vi "Reactor Write Client.vi"() -> ()   [LabVIEW 2017]
uses:
  <vilib>/OPCUA/controls/Write Status.ctl
  <vilib>/OPCUA/controls/NodeId.ctl
  <vilib>/OPCUA/client/Multiple Write Double Array.vi
  <vilib>/OPCUA/client/Multiple Write Bool Array.vi
  <vilib>/OPCUA/NI OPC UA Client.lvlib
panel:
  in  "error in (no error)":errorcluster
  in  "Stop Reactor Digital Control":bool
  in  "Node Status":T1 items=["Good"=0, "Uncertain_InitialValue"=1083310080, "Uncertain_LastUsableValue"=1083179008, "Uncertain_SensorNotAccurate"=1083375616, "Uncertain_EngineeringUnitsExceeded"=1083441152, "Bad_NoCommunication"=2150694912, "Bad_NotReadable"=2151284736, "Bad_NotWritable"=2151350272, "Bad_OutOfRange"=2151415808, "Bad_WaitingForInitialData"=2150760448]
  in  "Time Stamp":timestamp
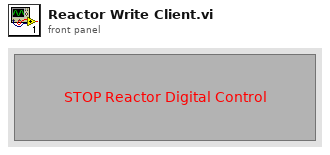
[diagram p1: front panel]
types:
  T1 = typedef "Write Status.ctl" = u32
  T2 = cluster{"message mode":enum16{"None", "Sign", "Sign and Encrypt"}, "security":enum16{"Basic256", "Basic128Rsa15"}}
  T3 = typedef "OPC UA Client Refnum.ctl" = refnum<k21>
  T4 = typedef "NodeId.ctl" = string
  T5 = cluster{"node ID":T4, "value":bool[], "timestamp (current time)":timestamp, "node status":T1}
  T6 = cluster{"node ID":T4, "value":dbl[], "timestamp (current time)":timestamp, "node status":T1}
  T7 = cluster{"node ID":T4, "value":dbl[], "timestamp (current time)":timestamp, "node status":T1}[]
  T8 = cluster{"node ID":T4, "value":bool[], "timestamp (current time)":timestamp, "node status":T1}[]
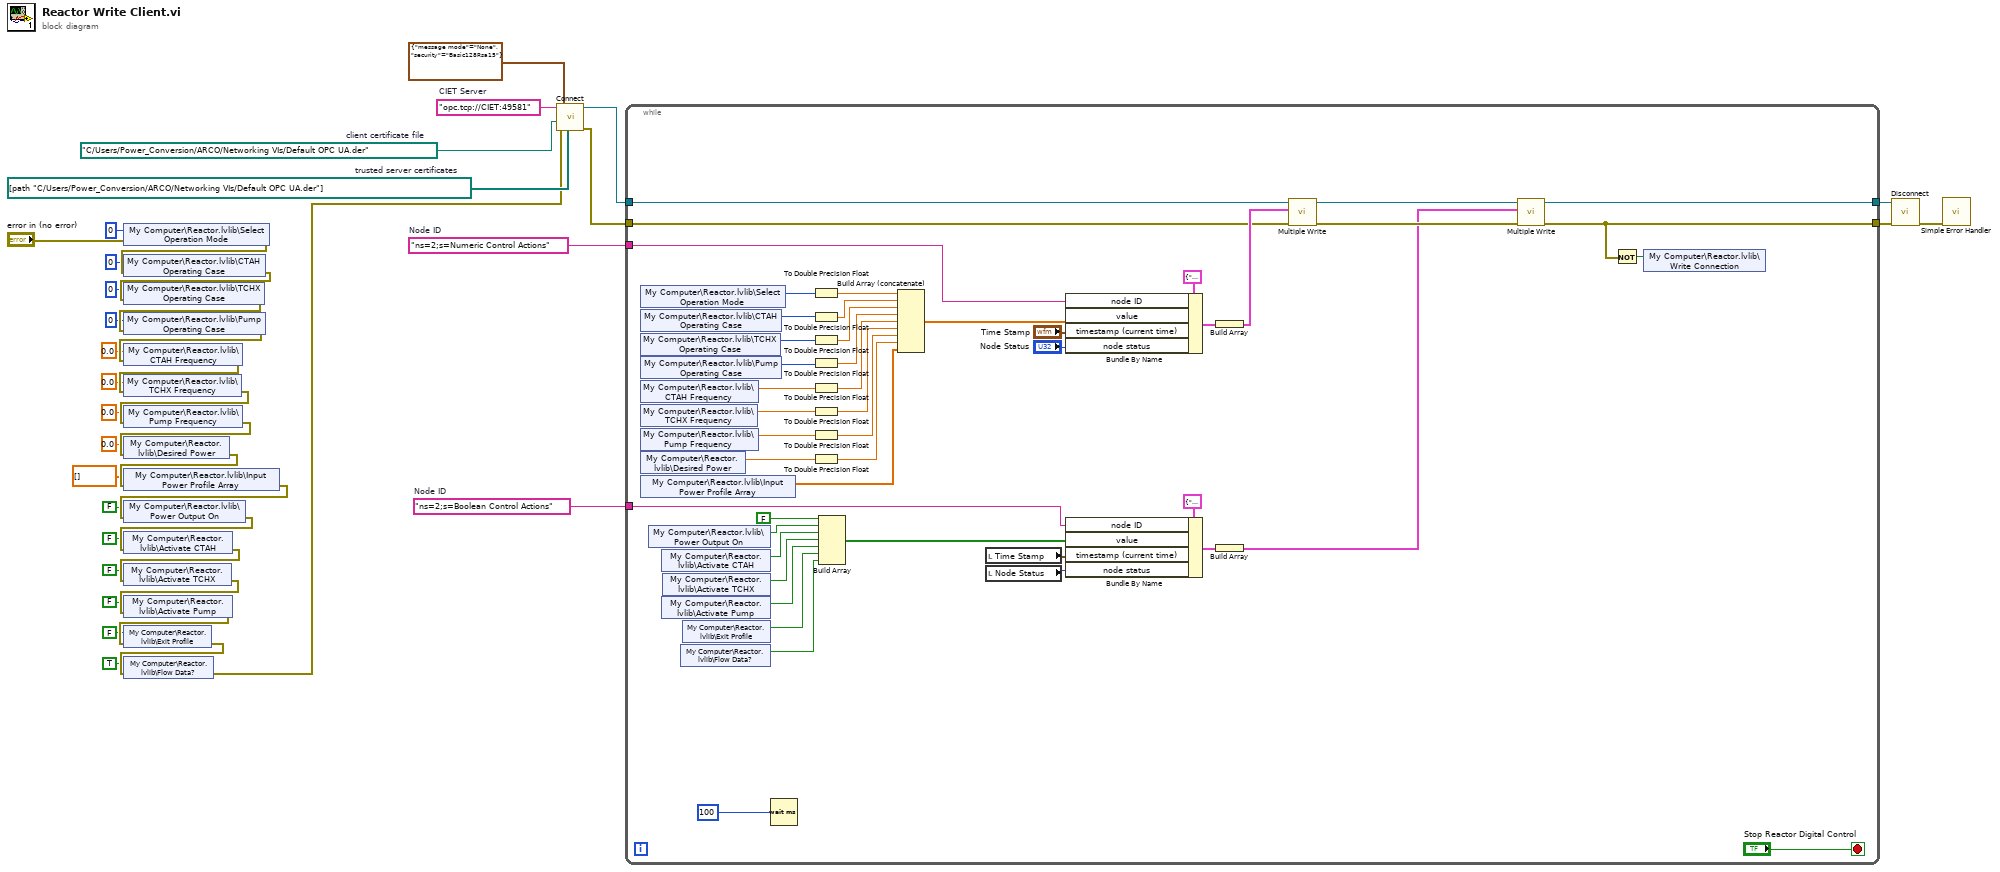
[diagram p0: block diagram]
diagram:
  w35 = "ns=2;s=Boolean Control Actions"  # Node ID
  w36 = "ns=2;s=Numeric Control Actions"  # Node ID
  w39 = path[] [path "C:/Users/Power_Conversion/ARCO/Networking VIs/Default OPC UA.der"]  # trusted server certificates
  w40 = path "C:/Users/Power_Conversion/ARCO/Networking VIs/Default OPC UA.der"  # client certificate file
  w42 = "opc.tcp://CIET:49581"  # CIET Server
  n1 = shared-variable "My Computer\\Reactor.lvlib\\Select Operation Mode"(u16 0 ("Select Operation Mode"), error in="error in (no error)") -> (error out=w30:errorcluster)
  n2 = shared-variable "My Computer\\Reactor.lvlib\\CTAH Operating Case"(0 ("CTAH Operating Case"), error in=w30) -> (error out=w29:errorcluster)
  n3 = shared-variable "My Computer\\Reactor.lvlib\\TCHX Operating Case"(0 ("TCHX Operating Case"), error in=w29) -> (error out=w28:errorcluster)
  n4 = shared-variable "My Computer\\Reactor.lvlib\\Pump Operating Case"(0 ("Pump Operating Case"), error in=w28) -> (error out=w27:errorcluster)
  n5 = shared-variable "My Computer\\Reactor.lvlib\\CTAH Frequency"(sgl 0.0 ("CTAH Frequency"), error in=w27) -> (error out=w26:errorcluster)
  n6 = shared-variable "My Computer\\Reactor.lvlib\\TCHX Frequency"(sgl 0.0 ("TCHX Frequency"), error in=w26) -> (error out=w25:errorcluster)
  n7 = shared-variable "My Computer\\Reactor.lvlib\\Pump Frequency"(sgl 0.0 ("Pump Frequency"), error in=w25) -> (error out=w24:errorcluster)
  n8 = shared-variable "My Computer\\Reactor.lvlib\\Desired Power"(sgl 0.0 ("Desired Power"), error in=w24) -> (error out=w23:errorcluster)
  n9 = shared-variable "My Computer\\Reactor.lvlib\\Input Power Profile Array"(dbl[] [] ("Input Power Profile Array"), error in=w23) -> (error out=w22:errorcluster)
  n10 = shared-variable "My Computer\\Reactor.lvlib\\Power Output On"(FALSE ("Power Output On"), error in=w22) -> (error out=w21:errorcluster)
  n11 = shared-variable "My Computer\\Reactor.lvlib\\Activate CTAH"(FALSE ("Activate CTAH"), error in=w21) -> (error out=w20:errorcluster)
  n12 = shared-variable "My Computer\\Reactor.lvlib\\Activate TCHX"(FALSE ("Activate TCHX"), error in=w20) -> (error out=w19:errorcluster)
  n13 = shared-variable "My Computer\\Reactor.lvlib\\Activate Pump"(FALSE ("Activate Pump"), error in=w19) -> (error out=w18:errorcluster)
  n14 = shared-variable "My Computer\\Reactor.lvlib\\Exit Profile"(FALSE ("Exit Profile"), error in=w18) -> (error out=w17:errorcluster)
  n15 = shared-variable "My Computer\\Reactor.lvlib\\Flow Data?"(TRUE ("Flow Data?"), error in=w17) -> (error out=w16:errorcluster)
  n16 = call <vilib>:"Connect.vi"("trusted server certificates"=w39, "error in (no error)"=w16, "client certificate file"=w40, "security policy"=T2 {"message mode"=enum."None", "security"=enum."Basic128Rsa15"}, "server endpoint URL"=w42) -> ("error out"=w37:errorcluster, "OPC UA client refnum out"=w38:T3)  [unwired: 4 in, 1 out]
  n17 = while {
    tunnel: w38 -> [w70]
    tunnel: w37 -> [w68]
    tunnel: w36 -> [w58]
    tunnel: w35 -> [w57]
    tunnel: [w54] -> w34
    tunnel: [w43] -> w33
    stop <- "Stop Reactor Digital Control" stop-if-true
    n18 = shared-variable "My Computer\\Reactor.lvlib\\Select Operation Mode"() -> (w89:u16)  [unwired: 1 in, 1 out]
    n19 = shared-variable "My Computer\\Reactor.lvlib\\CTAH Operating Case"() -> (w86:i32)  [unwired: 1 in, 1 out]
    n20 = shared-variable "My Computer\\Reactor.lvlib\\TCHX Operating Case"() -> (w87:i32)  [unwired: 1 in, 1 out]
    n21 = shared-variable "My Computer\\Reactor.lvlib\\Pump Operating Case"() -> (w88:i32)  [unwired: 1 in, 1 out]
    n22 = shared-variable "My Computer\\Reactor.lvlib\\CTAH Frequency"() -> (w53:sgl)  [unwired: 1 in, 1 out]
    n23 = shared-variable "My Computer\\Reactor.lvlib\\TCHX Frequency"() -> (w52:sgl)  [unwired: 1 in, 1 out]
    n24 = shared-variable "My Computer\\Reactor.lvlib\\Pump Frequency"() -> (w51:sgl)  [unwired: 1 in, 1 out]
    n25 = shared-variable "My Computer\\Reactor.lvlib\\Desired Power"() -> (w50:sgl)  [unwired: 1 in, 1 out]
    n26 = shared-variable "My Computer\\Reactor.lvlib\\Input Power Profile Array"() -> (w45:dbl[])  [unwired: 1 in, 1 out]
    n27 = shared-variable "My Computer\\Reactor.lvlib\\Power Output On"() -> (w80:bool)  [unwired: 1 in, 1 out]
    n28 = shared-variable "My Computer\\Reactor.lvlib\\Activate CTAH"() -> (w79:bool)  [unwired: 1 in, 1 out]
    n29 = shared-variable "My Computer\\Reactor.lvlib\\Activate Pump"() -> (w77:bool)  [unwired: 1 in, 1 out]
    n30 = shared-variable "My Computer\\Reactor.lvlib\\Activate TCHX"() -> (w78:bool)  [unwired: 1 in, 1 out]
    n31 = shared-variable "My Computer\\Reactor.lvlib\\Flow Data?"() -> (w75:bool)  [unwired: 1 in, 1 out]
    n32 = shared-variable "My Computer\\Reactor.lvlib\\Exit Profile"() -> (w76:bool)  [unwired: 1 in, 1 out]
    n33 = Wait (ms)(milliseconds to wait=u32 100) -> ()  [unwired: 1 out]
    n34 = To Double Precision Float(number=w89) -> (double precision float=w85:dbl)
    n35 = To Double Precision Float(number=w86) -> (double precision float=w84:dbl)
    n36 = To Double Precision Float(number=w87) -> (double precision float=w83:dbl)
    n37 = To Double Precision Float(number=w88) -> (double precision float=w82:dbl)
    n38 = To Double Precision Float(number=w53) -> (double precision float=w49:dbl)
    n39 = To Double Precision Float(number=w52) -> (double precision float=w48:dbl)
    n40 = To Double Precision Float(number=w51) -> (double precision float=w47:dbl)
    n41 = To Double Precision Float(number=w50) -> (double precision float=w46:dbl)
    n42 = Build Array(FALSE, w80, w79, w78, w77, w76, w75) -> (w63:bool[])
    n43 = Build Array (concatenate)(w85, w84, w83, w82, w49, w48, w47, w46, w45) -> (w73:dbl[])
    n44 = local read "Time Stamp"() -> (w60:timestamp)
    n45 = local read "Node Status"() -> (w59:T1)
    n46 = Bundle By Name(cluster=T6 {"node ID"="", "value"=[], "timestamp (current time)"=timestamp(0 s since 1904-01-01), "node status"=0} ("request"), "node ID"=w58, "value"=w73, "timestamp (current time)"="Time Stamp", "node status"="Node Status") -> (w72:T6)
    n47 = Bundle By Name(cluster=T5 {"node ID"="", "value"=[], "timestamp (current time)"=timestamp(0 s since 1904-01-01), "node status"=0} ("request"), "node ID"=w57, "value"=w63, "timestamp (current time)"=w60, "node status"=w59) -> (w65:T5)
    n48 = Build Array(w72) -> (w71:T7)
    n49 = Build Array(w65) -> (w64:T8)
    n50 = call-poly <vilib>:"Multiple Write.vi"("error in (no error)"=w68, "requests"=w71, "OPC UA client refnum in"=w70) -> ("error out"=w67:errorcluster, "OPC UA client refnum out"=w69:T3)  [unwired: 5 in, 2 out]
    n51 = call-poly <vilib>:"Multiple Write.vi"("error in (no error)"=w67, "requests"=w64, "OPC UA client refnum in"=w69) -> ("error out"=w43:errorcluster, "OPC UA client refnum out"=w54:T3)  [unwired: 5 in, 2 out]
    n52 = Not(x=w43) -> (.not. x?=w44:bool)
    n53 = shared-variable "My Computer\\Reactor.lvlib\\Write Connection"(w44) -> ()  [unwired: 1 in, 1 out]
  }
  n54 = call <vilib>:"Disconnect.vi"("error in (no error)"=w33, "OPC UA client refnum in"=w34) -> ("error out"=w32:errorcluster)  [unwired: 9 in]
  n55 = call <vilib>:"Simple Error Handler.vi"("error in (no error)"=w32) -> ()  [unwired: 4 in, 5 out]
